vi "Get Device Info.vi"(8 "error in (no error)":errorcluster, 11 "RIO Device":T1) -> (0 "error out":errorcluster, 1 "SI Channels":string[](array[string]), 2 "SI Count":i32, 3 "Module Name":string)   [LabVIEW 2025, in "I2C Bus Monitor UI.lvlib"]
uses:
  I2C Bus Monitor UI.lvlib
  <vilib>/userDefined/Silver/nirio_resource_slv.ctl
  <vilib>/nisyscfg/Close (Filter).vi
  <vilib>/nisyscfg/Close (System).vi
  <vilib>/nisyscfg/Close (Hardware).vi
  I2C UI Error Strings Global.vi
  <vilib>/nisyscfg/nisyscfg.lvlib
  <resource>/objmgr/niflexrioatomicsae.rc
  <resource>/objmgr/nicriosae.rc
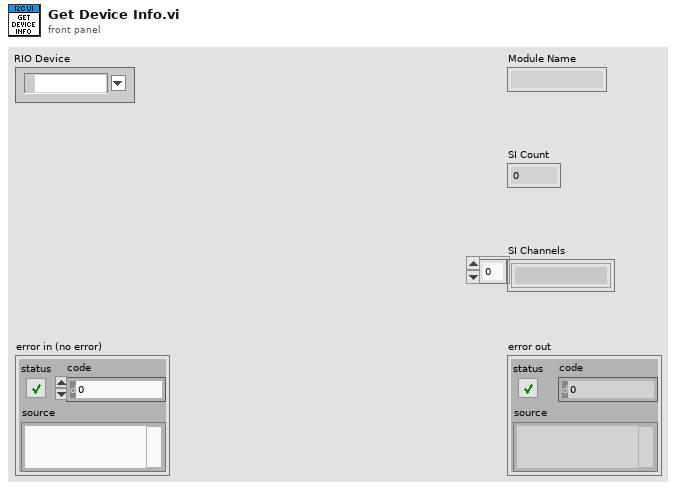
[diagram p1: front panel]
types:
  T1 = typedef "nirio_resource_slv.ctl" = tag
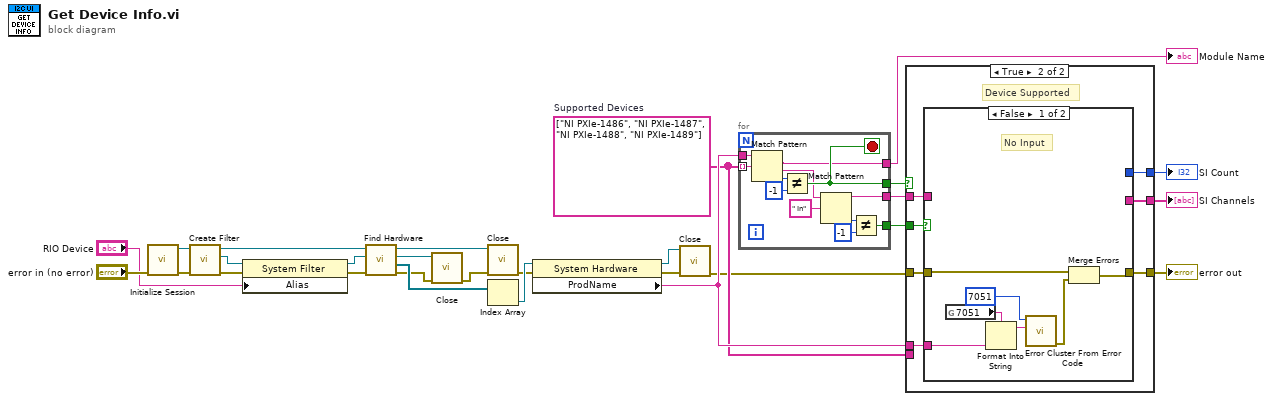
[diagram p0: block diagram]
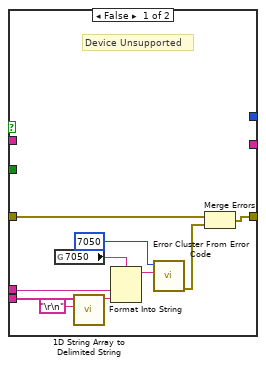
[diagram p2: hidden frame]
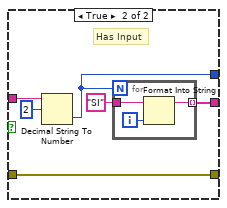
[diagram p3: hidden frame]
diagram:
  w7 = string[] ["NI PXIe-1486", "NI PXIe-1487", "NI PXIe-1488", "NI PXIe-1489"]  # Supported Devices
  n1 = call <vilib>:"Initialize Session.vi"("error in (no error)"="error in (no error)") -> ("error out"=w19:errorcluster, "Session out"=w17:refnum<k21>)  [unwired: 9 in]
  n2 = call <vilib>:"Create Filter.vi"("error in (no error)"=w19, "Session in"=w17) -> ("error out"=w14:errorcluster, "Filter out"=w15:refnum<k20>, "Session out"=w18:refnum<k21>)  [unwired: 7 in]
  n3 = property class="System Filter"(reference=w15, error in=w14, "Alias"="RIO Device") -> (reference out=w16:refnum<k20>, error out=w20:errorcluster)
  n4 = call <vilib>:"Find Hardware.vi"("error in (no error)"=w20, "Filter in"=w16, "Session in"=w18) -> ("error out"=w3:errorcluster, "Resources out"=w13:refnum<k20>[], "Filter out"=w2:refnum<k20>, "Session out"=w12:refnum<k21>)  [unwired: 5 in]
  n5 = call-poly <vilib>:"Close.vi"("error in (no error)"=w3, "Filter in"=w2) -> ("error out"=w1:errorcluster)  [unwired: 9 in]
  n6 = call-poly <vilib>:"Close.vi"("error in (no error)"=w1, "Session in"=w12) -> ("error out"=w11:errorcluster)  [unwired: 9 in]
  n7 = Index Array(array=w13) -> (element=w22:refnum<k20>)  [unwired: 1 in]
  n8 = property class="System Hardware"(reference=w22, error in=w11) -> (reference out=w6:refnum<k20>, error out=w5:errorcluster, "ProdName"=w8:string)
  n9 = call-poly <vilib>:"Close.vi"("error in (no error)"=w5, "Resource in"=w6) -> ("error out"=w4:errorcluster)  [unwired: 9 in]
  n10 = for {
    tunnel: w7 -> [w34] mode=indexing
    tunnel: w8 -> [w40]
    tunnel: [w37] -> w10
    tunnel: [w33] -> w26
    tunnel: [w31] -> w23
    tunnel: [w30] -> w25
    stop <- w37 stop-if-true
    n11 = Match Pattern(string=w40, regular expression=w34) -> (match substring=w33:string, after substring=w29:string, offset past match=w39:i32)  [unwired: 1 in, 1 out]
    n12 = Not Equal?(x=w39, y=-1) -> (x != y?=w37:bool)
    n13 = Match Pattern(string=w29, regular expression=" In") -> (before substring=w31:string, offset past match=w35:i32)  [unwired: 1 in, 2 out]
    n14 = Not Equal?(x=w35, y=-1) -> (x != y?=w30:bool)
  }
  "Module Name" <- w26
  n15 = case shown="True" w10 {
    tunnel: [_ w57] -> w27
    tunnel: w25 -> [_ w56]
    tunnel: [_ w55] -> w24
    tunnel: w23 -> [_ w54]
    tunnel: w4 -> [w43 w53]
    tunnel: [w42 w52] -> w9
    tunnel: w8 -> [w49 w51]
    tunnel: w7 -> [w48 _]
    frame False {
      # "Device Unsupported"
      n16 = global read "I2C UI Error Strings Global.vi" "7050"() -> (w50:string)
      n17 = call <vilib>:"1D String Array to Delimited String.vi"("delimiter"="\r\n", "string array"=w48) -> ("delimited string"=w46:string)  [unwired: 9 in]
      n18 = Format Into String(format string=w50, w49, w46) -> (resulting string=w45:string)  [unwired: 2 in, 1 out]
      n19 = call <vilib>:"Error Cluster From Error Code.vi"("error message (\"\")"=w45, "error code (0)"=7050) -> ("error out"=w41:errorcluster)  [unwired: 7 in]
      n20 = Merge Errors(w43, w41) -> (w42:errorcluster)
    }
    frame True {
      # "Device Supported"
      n21 = case shown="False" w56 {
        tunnel: w54 -> [_ w70]
        tunnel: [_ w68] -> w57
        tunnel: [_ w66] -> w55
        tunnel: w53 -> [w59 w65]
        tunnel: [w58 w65] -> w52
        tunnel: w51 -> [w60 _]
        frame False {
          # "No Input"
          n22 = global read "I2C UI Error Strings Global.vi" "7051"() -> (w64:string)
          n23 = Format Into String(format string=w64, w60) -> (resulting string=w63:string)  [unwired: 2 in, 1 out]
          n24 = call <vilib>:"Error Cluster From Error Code.vi"("error message (\"\")"=w63, "error code (0)"=7051) -> ("error out"=w61:errorcluster)  [unwired: 7 in]
          n25 = Merge Errors(w59, w61) -> (w58:errorcluster)
        }
        frame True {
          # "Has Input"
          n26 = Decimal String To Number(string=w70, offset=2) -> (number=w68:i32)  [unwired: 1 in, 1 out]
          n27 = for {
            N: w68 -> [_]
            tunnel: "SI" -> [w73]
            tunnel: [w71] -> w66 mode=indexing
            i -> [w72]
            n28 = Format Into String(initial string=w73, w72) -> (resulting string=w71:string)  [unwired: 2 in, 1 out]
          }
        }
      }
    }
  }
  "error out" <- w9
  "SI Count" <- w27
  "SI Channels" <- w24
